vi "variant to tree helper.vi"(4 "is array element?":bool, 5 "is attribute?":bool, 6 "index string":string, 7 "name":string, 8 "error in (no error)":errorcluster, 9 "Item Indent":i32, 10 "Variant":variant, 11 "Items":T1(array[cluster])) -> (0 "error out":errorcluster, 3 "Items out":T1(array[cluster]))   [LabVIEW 2016]
uses:
  <vilib>/Utility/Data Type/NI_Data Type.lvlib
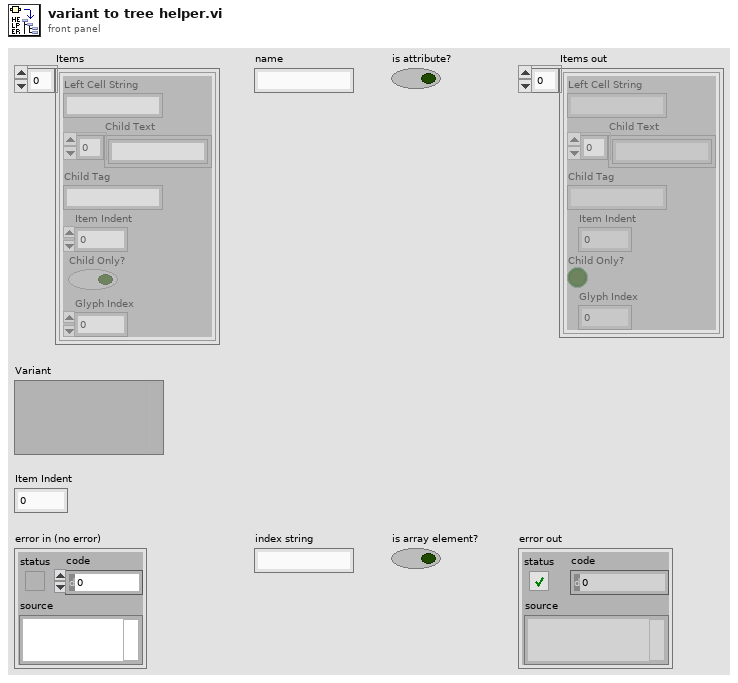
[diagram p1: front panel]
types:
  T1 = cluster{"Left Cell String":string, "Child Text":string[], "Child Tag":string, "Item Indent":i32, "Child Only?":bool, "Glyph Index":i32}[]
  T2 = typedef "NI_Data Type.lvlib/Data Type.ctl" = enum8{"Invalid Type", "Void", "I8", "I16", "I32", "I64", "U8", "U16", "U32", "U64", "Single Float", "Double Float", "Extended Float", "Single Complex", "Double Complex", "Extended Complex", "Enum U8", "Enum U16", "Enum U32", "Enum U64", "Single Float With Unit", "Double Float With Unit", "Extended Float With Unit", "Single Complex with Unit", "Double Complex with Unit", "Extended Complex with Unit", "Boolean", "String", "Path", "Picture", "Tag", "Array", "Cluster", "Variant", "LV Variant", "Waveform", "Timestamp", "Digital Waveform", "Digital Data", "ExpressData", "Refnum", "External Data", "VI", "Poly VI", "LabVIEW Class Instance", "Fixed Point"}
  T3 = cluster{"Left Cell String":string, "Child Text":string[], "Child Tag":string, "Item Indent":i32, "Child Only?":bool, "Glyph Index":i32}
  T4 = typedef "LVFixedPointRepRangeTypeDef.ctl" = cluster{"Range Min":dbl, "Range Max":dbl, "Delta":dbl}
  T5 = typedef "LVFixedPointRepBitsTypeDef.ctl" = cluster{"Signed":bool, "Word Length":u32, "Integer Word Length":i32}
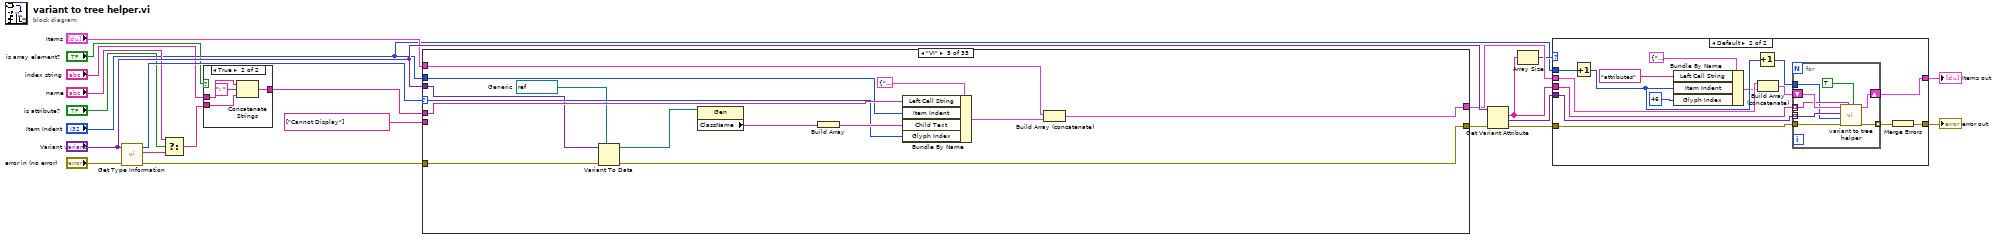
[diagram p0: block diagram]
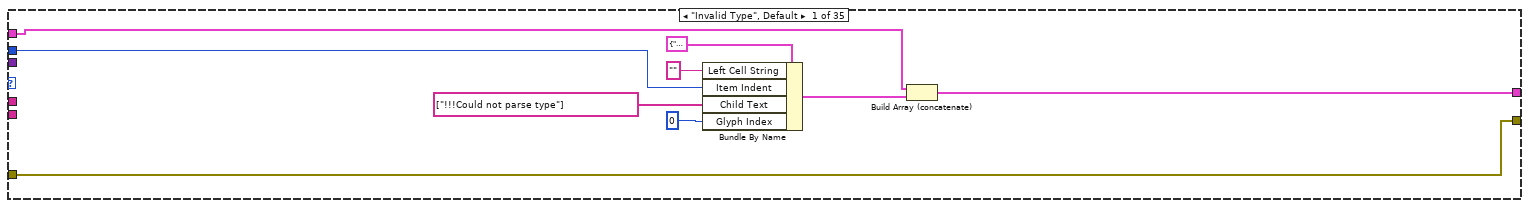
[diagram p4: hidden frame]
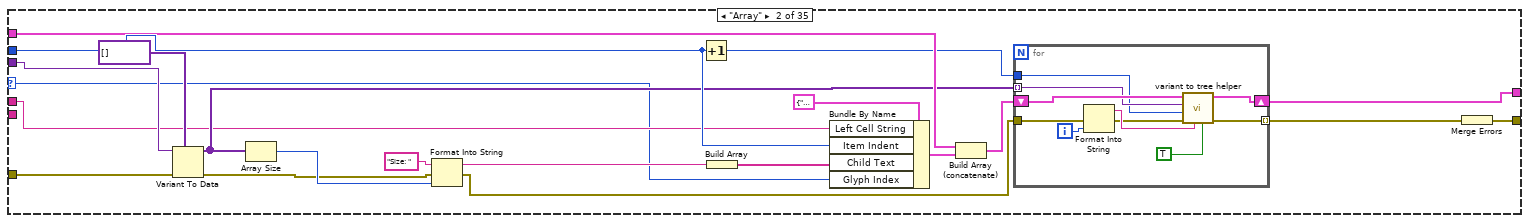
[diagram p5: hidden frame]
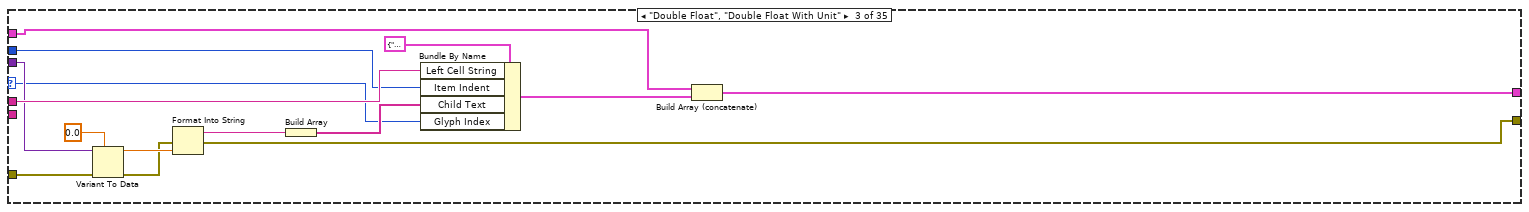
[diagram p6: hidden frame]
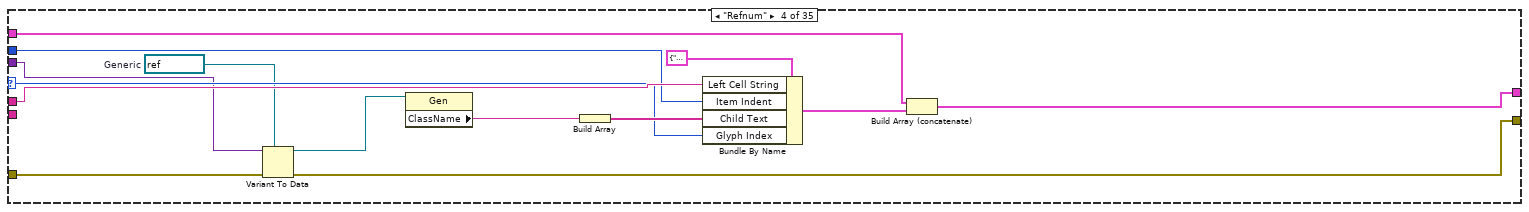
[diagram p7: hidden frame]
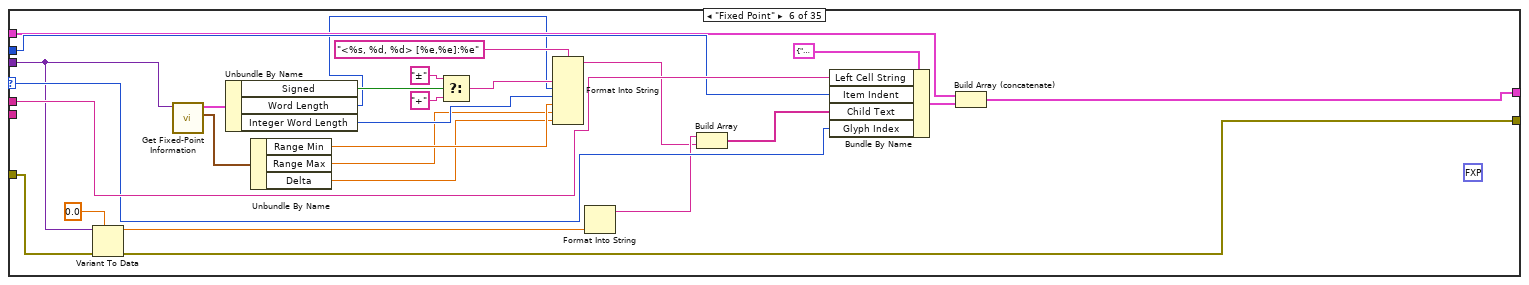
[diagram p8: hidden frame]
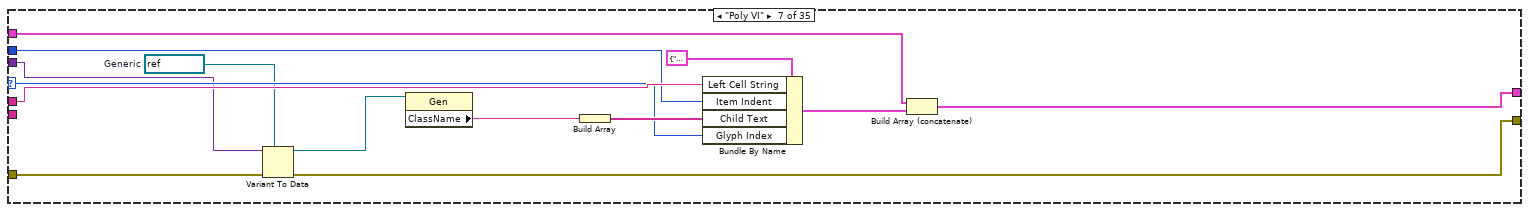
[diagram p9: hidden frame]
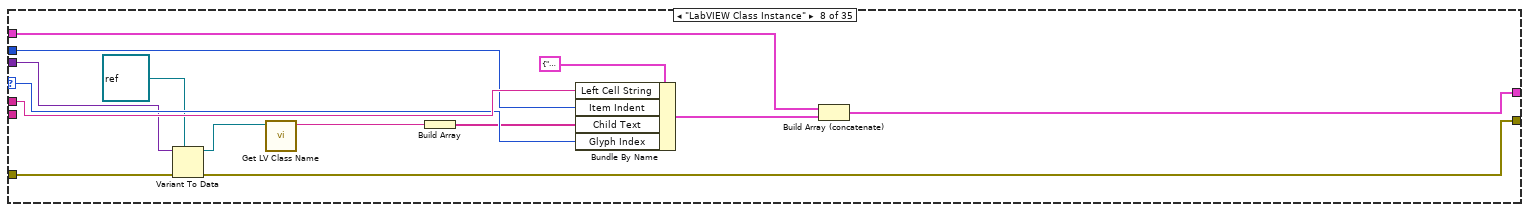
[diagram p10: hidden frame]
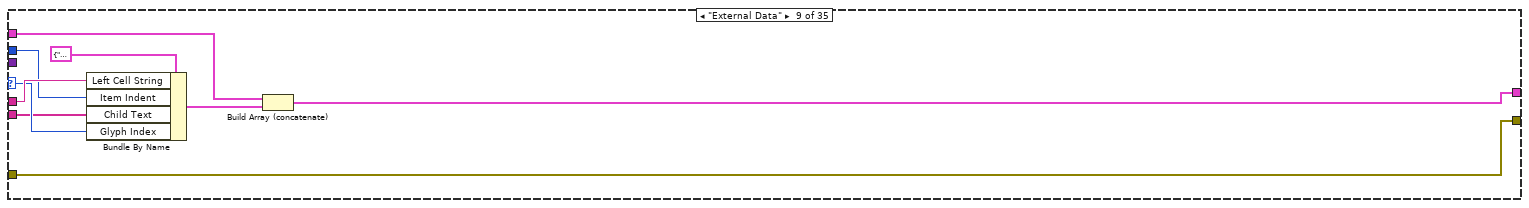
[diagram p11: hidden frame]
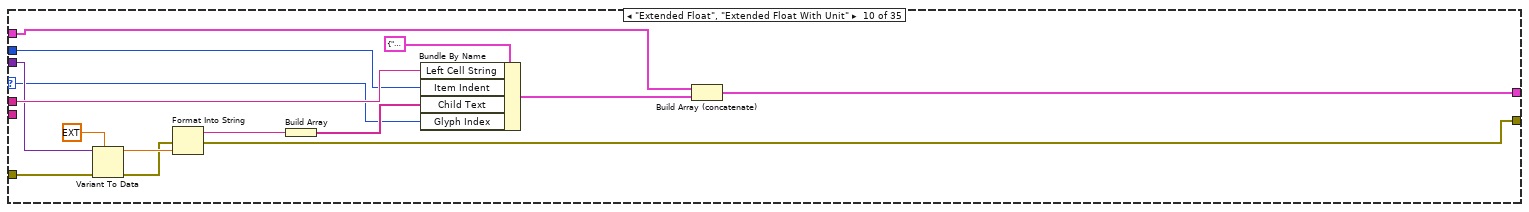
[diagram p12: hidden frame]
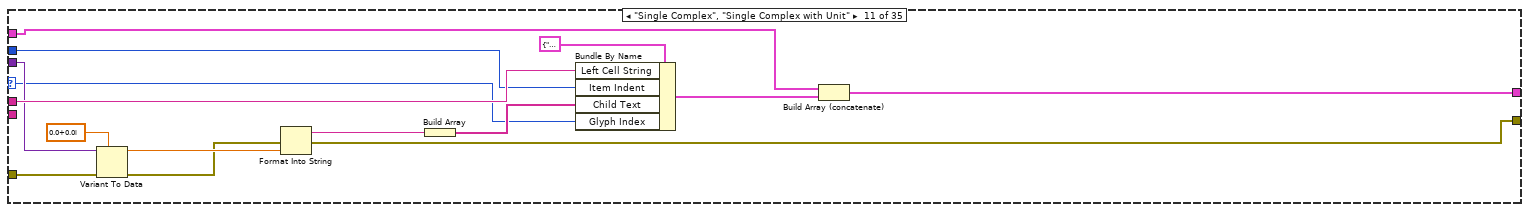
[diagram p13: hidden frame]
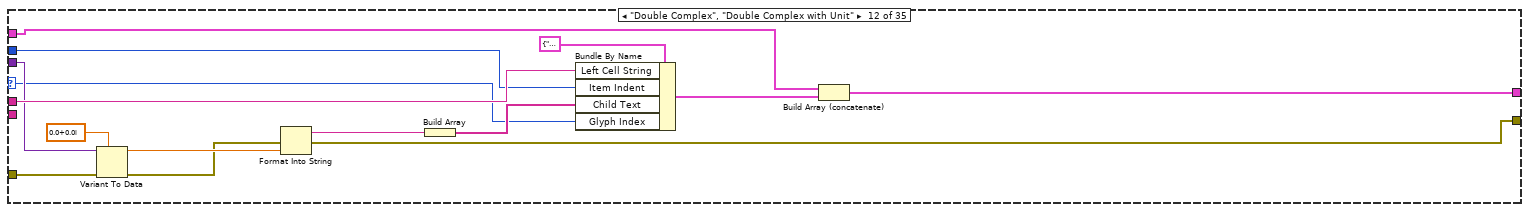
[diagram p14: hidden frame]
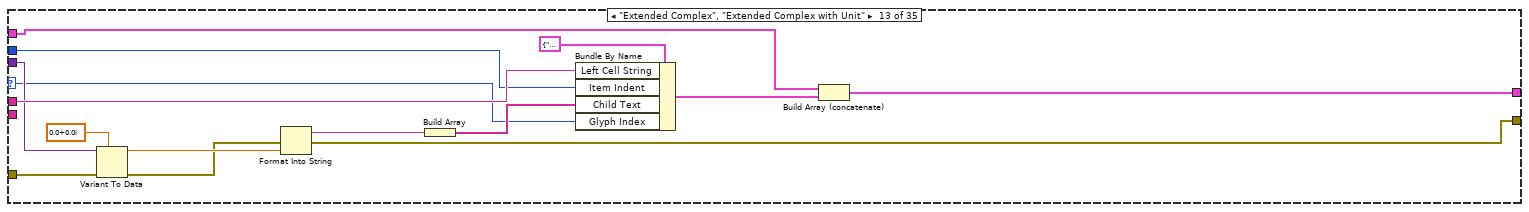
[diagram p15: hidden frame]
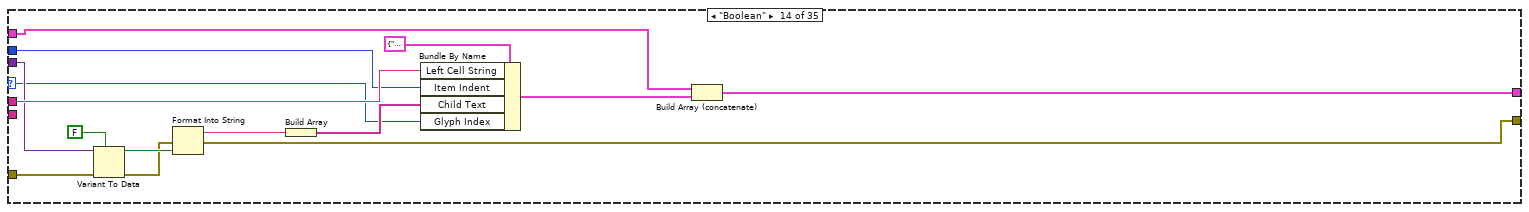
[diagram p16: hidden frame]
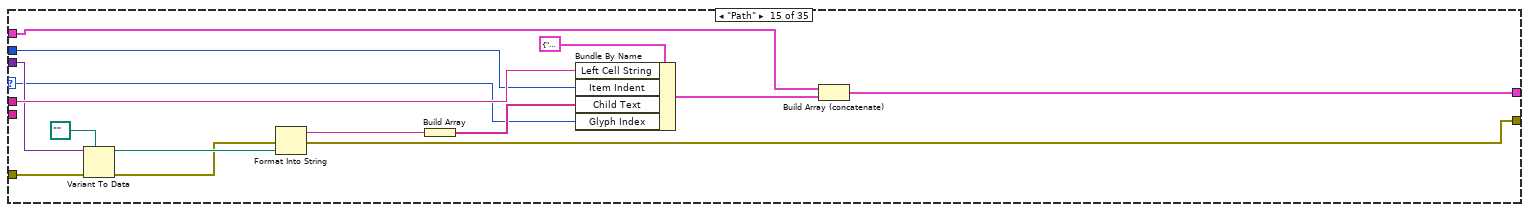
[diagram p17: hidden frame]
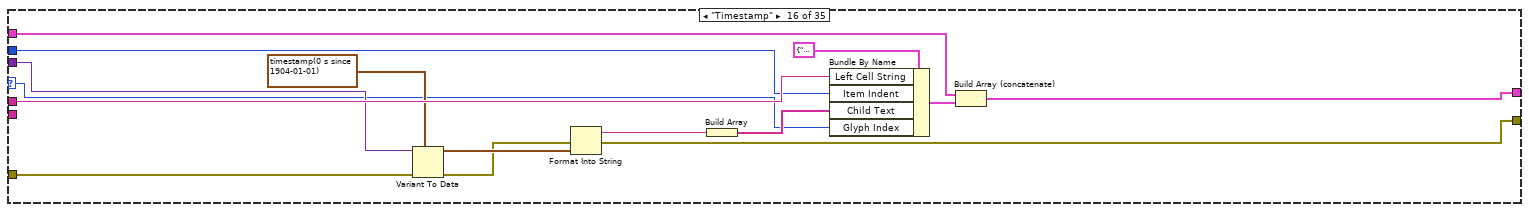
[diagram p18: hidden frame]
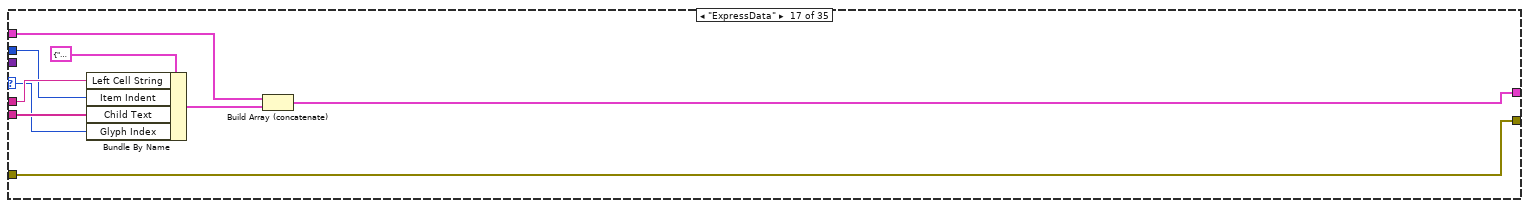
[diagram p19: hidden frame]
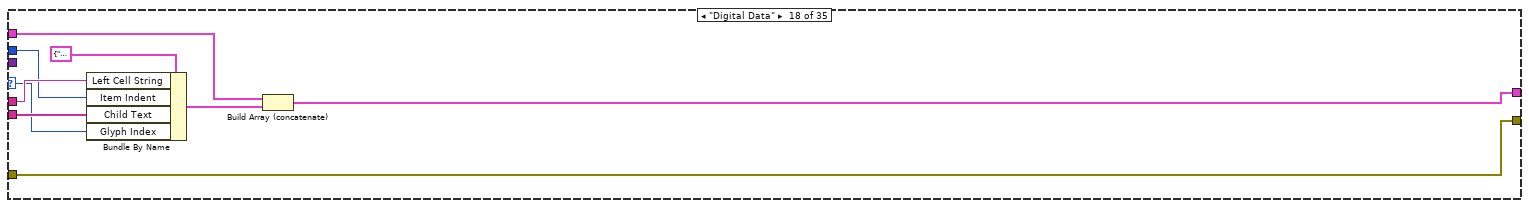
[diagram p20: hidden frame]
diagram:
  n1 = call <vilib>:"Get Type Information.vi"("error in (no error)"="error in (no error)", "Variant"="Variant") -> ("error out"=w4:errorcluster, "Name"=w14:string, "Type"=w22:T2)  [unwired: 5 in, 2 out]
  n2 = Select(t="name", s="is attribute?", f=w14) -> (s? t:f=w7:string)
  n3 = case shown="True" "is array element?" {
    tunnel: "index string" -> [_ w27]
    tunnel: w7 -> [w23 w25]
    tunnel: [w23 w24] -> w6
    frame False {
    }
    frame True {
      n4 = Concatenate Strings(w27, ": " ("string"), w25) -> (w24:string)
    }
  }
  n5 = case shown="\"VI\"" w22 {
    selector: w22 -> [_ w42 w71 w89 w103 w131 w144 w159 w168 w178 w193 w208 w223 w238 w253 w268 w281 w290 w299 w308 w317 w330 w361 w370 w380 w393 w409 w424 w439 w454 w469 w484 w499 w514 w529]
    tunnel: "Items" -> [w30 w53 w74 w92 w106 w134 w147 w162 w171 w181 w196 w211 w226 w241 w256 w271 w285 w294 w303 w313 w321 w344 w365 w374 w383 w401 w416 w431 w446 w461 w476 w491 w506 w521 w536]
    tunnel: "Variant" -> [_ w57 w79 w86 w100 w127 w141 w156 _ w186 w201 w216 w231 w246 w261 w276 _ _ _ _ _ w332 _ _ w387 w398 w413 w428 w443 w458 w473 w488 w503 w518 w533]
    tunnel: w6 -> [_ w43 w81 w95 w109 w136 w150 w164 w173 w188 w203 w218 w233 w248 w263 w278 w287 w296 w305 w314 w323 w345 w367 w376 w389 w404 w419 w434 w449 w464 w479 w494 w509 w524 w539]
    tunnel: "Item Indent" -> [w33 w54 w80 w94 w108 w135 w149 w163 w172 w187 w202 w217 w232 w247 w262 w277 w286 w295 w304 w309 w322 w339 w366 w375 w388 w403 w418 w433 w448 w463 w478 w493 w508 w523 w538]
    tunnel: [w28 w49 w72 w90 w104 w132 w145 w160 w169 w179 w194 w209 w224 w239 w254 w269 w283 w292 w301 w310 w319 w340 w363 w372 w381 w399 w414 w429 w444 w459 w474 w489 w504 w519 w534] -> w17
    tunnel: string[] ["Cannot Display"] ("Child Text") -> [_ _ _ _ _ _ _ _ w166 _ _ _ _ _ _ _ w282 w291 w300 w311 w318 _ w362 w371 _ _ _ _ _ _ _ _ _ _ _]
    tunnel: w4 -> [w36 w41 w70 w88 w102 w130 w143 w158 w167 w177 w192 w207 w222 w237 w252 w267 w280 w289 w298 w307 w316 w329 w360 w369 w379 w392 w408 w423 w438 w453 w468 w483 w498 w513 w528]
    tunnel: [w36 w37 w68 w87 w101 w129 w142 w157 w167 w175 w190 w205 w220 w235 w250 w265 w280 w289 w298 w307 w316 w325 w360 w369 w378 w391 w406 w421 w436 w451 w466 w481 w496 w511 w526] -> w1
    frame "Invalid Type", Default {
      n6 = Bundle By Name(cluster=T3 {"Left Cell String"="", "Child Text"=[], "Child Tag"="", "Item Indent"=0, "Child Only?"=FALSE, "Glyph Index"=0} ("Item"), "Left Cell String"="", "Item Indent"=w33, "Child Text"=string[] ["!!!Could not parse type"], "Glyph Index"=0) -> (w29:T3)
      n7 = Build Array (concatenate)(w30, w29) -> (w28:T1)
    }
    frame "Array" {
      n8 = Variant To Data(error in=w41, type=variant[] [], Variant=w57) -> (data=w47:variant[], error out=w40:errorcluster)
      n9 = Array Size(array=w47) -> (size(s)=w46:i32)
      n10 = Format Into String(initial string="Size: " ("string"), error in=w40, w46) -> (resulting string=w45:string, error out=w39:errorcluster)  [unwired: 1 in]
      n11 = Increment(x=w54) -> (x+1=w48:i32)
      n12 = Build Array(w45) -> (w51:string[])
      n13 = Bundle By Name(cluster=T3 {"Left Cell String"="", "Child Text"=[], "Child Tag"="", "Item Indent"=0, "Child Only?"=FALSE, "Glyph Index"=0} ("Item"), "Left Cell String"=w43, "Item Indent"=w54, "Child Text"=w51, "Glyph Index"=w42) -> (w52:T3)
      n14 = Build Array (concatenate)(w53, w52) -> (w50:T1)
      n15 = for {
        tunnel: w47 -> [w65] mode=indexing
        shift-right: [w66] -> w49
        shift-left: w50 -> [w67]
        tunnel: w48 -> [w64]
        tunnel: w39 -> [w60]
        tunnel: [w58] -> w38 mode=indexing
        i -> [w63]
        n16 = Format Into String(error in=w60, w63) -> (resulting string=w62:string, error out=w59:errorcluster)  [unwired: 2 in]
        n17 = call "variant to tree helper.vi"("is array element?"=TRUE, "index string"=w62, "error in (no error)"=w59, "Item Indent"=w64, "Variant"=w65, "Items"=w67) -> ("error out"=w58:errorcluster, "Items out"=w66:T1)  [unwired: 4 in]
      }
      n18 = Merge Errors(w38) -> (w37:errorcluster)
    }
    frame "Double Float", "Double Float With Unit" {
      n19 = Variant To Data(error in=w70, type=0.0, Variant=w79) -> (data=w77:dbl, error out=w69:errorcluster)
      n20 = Format Into String(error in=w69, w77) -> (resulting string=w76:string, error out=w68:errorcluster)  [unwired: 2 in]
      n21 = Build Array(w76) -> (w75:string[])
      n22 = Bundle By Name(cluster=T3 {"Left Cell String"="", "Child Text"=[], "Child Tag"="", "Item Indent"=0, "Child Only?"=FALSE, "Glyph Index"=0} ("Item"), "Left Cell String"=w81, "Item Indent"=w80, "Child Text"=w75, "Glyph Index"=w71) -> (w73:T3)
      n23 = Build Array (concatenate)(w74, w73) -> (w72:T1)
    }
    frame "Refnum" {
      w85 = refnum<vi> refnum  # Generic
      n24 = Variant To Data(error in=w88, type=w85, Variant=w86) -> (data=w84:refnum<vi>, error out=w87:errorcluster)
      n25 = property class="Gen"(reference=w84) -> ("ClassName"=w83:string)  [unwired: 1 in, 2 out]
      n26 = Build Array(w83) -> (w93:string[])
      n27 = Bundle By Name(cluster=T3 {"Left Cell String"="", "Child Text"=[], "Child Tag"="", "Item Indent"=0, "Child Only?"=FALSE, "Glyph Index"=0} ("Item"), "Left Cell String"=w95, "Item Indent"=w94, "Child Text"=w93, "Glyph Index"=w89) -> (w91:T3)
      n28 = Build Array (concatenate)(w92, w91) -> (w90:T1)
    }
    frame "VI" {
      w99 = refnum<vi> refnum  # Generic
      n29 = Variant To Data(error in=w102, type=w99, Variant=w100) -> (data=w98:refnum<vi>, error out=w101:errorcluster)
      n30 = property class="Gen"(reference=w98) -> ("ClassName"=w97:string)  [unwired: 1 in, 2 out]
      n31 = Build Array(w97) -> (w107:string[])
      n32 = Bundle By Name(cluster=T3 {"Left Cell String"="", "Child Text"=[], "Child Tag"="", "Item Indent"=0, "Child Only?"=FALSE, "Glyph Index"=0} ("Item"), "Left Cell String"=w109, "Item Indent"=w108, "Child Text"=w107, "Glyph Index"=w103) -> (w105:T3)
      n33 = Build Array (concatenate)(w106, w105) -> (w104:T1)
    }
    frame "Fixed Point" {
      (unwired) fxp<+,1,1> 0.0
      n34 = Variant To Data(error in=w130, type=0.0, Variant=w127) -> (data=w126:dbl, error out=w129:errorcluster)
      n35 = call <vilib>:"Get Fixed-Point Information.vi"("Variant"=w127) -> ("FXP Range"=w116:T4, "FXP Representation"=w123:T5)  [unwired: 7 in, 2 out]
      n36 = Unbundle By Name(w123) -> ("Signed"=w122:bool, "Word Length"=w118:u32, "Integer Word Length"=w117:i32)
      n37 = Unbundle By Name(w116) -> ("Range Min"=w115:dbl, "Range Max"=w114:dbl, "Delta"=w113:dbl)
      n38 = Select(t="±", s=w122, f="+" ("format string")) -> (s? t:f=w119:string)
      n39 = Format Into String(format string="<%s, %d, %d> [%e,%e]:%e", w119, w118, w117, w115, w114, w113) -> (resulting string=w111:string)  [unwired: 2 in, 1 out]
      n40 = Format Into String(w126) -> (resulting string=w125:string)  [unwired: 3 in, 1 out]
      n41 = Build Array(w125, w111) -> (w112:string[])
      n42 = Bundle By Name(cluster=T3 {"Left Cell String"="", "Child Text"=[], "Child Tag"="", "Item Indent"=0, "Child Only?"=FALSE, "Glyph Index"=0} ("Item"), "Left Cell String"=w136, "Item Indent"=w135, "Child Text"=w112, "Glyph Index"=w131) -> (w133:T3)
      n43 = Build Array (concatenate)(w134, w133) -> (w132:T1)
    }
    frame "Poly VI" {
      w140 = refnum<vi> refnum  # Generic
      n44 = Variant To Data(error in=w143, type=w140, Variant=w141) -> (data=w139:refnum<vi>, error out=w142:errorcluster)
      n45 = property class="Gen"(reference=w139) -> ("ClassName"=w138:string)  [unwired: 1 in, 2 out]
      n46 = Build Array(w138) -> (w148:string[])
      n47 = Bundle By Name(cluster=T3 {"Left Cell String"="", "Child Text"=[], "Child Tag"="", "Item Indent"=0, "Child Only?"=FALSE, "Glyph Index"=0} ("Item"), "Left Cell String"=w150, "Item Indent"=w149, "Child Text"=w148, "Glyph Index"=w144) -> (w146:T3)
      n48 = Build Array (concatenate)(w147, w146) -> (w145:T1)
    }
    frame "LabVIEW Class Instance" {
      n49 = Variant To Data(error in=w158, type=refnum<class> refnum ("LabVIEW Object"), Variant=w156) -> (data=w154:refnum<class>, error out=w157:errorcluster)
      n50 = call <vilib>:"Get LV Class Name.vi"("object"=w154) -> ("class name"=w153:string)  [unwired: 9 in, 1 out]
      n51 = Build Array(w153) -> (w152:string[])
      n52 = Bundle By Name(cluster=T3 {"Left Cell String"="", "Child Text"=[], "Child Tag"="", "Item Indent"=0, "Child Only?"=FALSE, "Glyph Index"=0} ("Item"), "Left Cell String"=w164, "Item Indent"=w163, "Child Text"=w152, "Glyph Index"=w159) -> (w161:T3)
      n53 = Build Array (concatenate)(w162, w161) -> (w160:T1)
    }
    frame "External Data" {
      n54 = Bundle By Name(cluster=T3 {"Left Cell String"="", "Child Text"=[], "Child Tag"="", "Item Indent"=0, "Child Only?"=FALSE, "Glyph Index"=0} ("Item"), "Left Cell String"=w173, "Item Indent"=w172, "Child Text"=w166, "Glyph Index"=w168) -> (w170:T3)
      n55 = Build Array (concatenate)(w171, w170) -> (w169:T1)
    }
    frame "Extended Float", "Extended Float With Unit" {
      n56 = Variant To Data(error in=w177, type=ext 0.0, Variant=w186) -> (data=w184:ext, error out=w176:errorcluster)
      n57 = Format Into String(error in=w176, w184) -> (resulting string=w183:string, error out=w175:errorcluster)  [unwired: 2 in]
      n58 = Build Array(w183) -> (w182:string[])
      n59 = Bundle By Name(cluster=T3 {"Left Cell String"="", "Child Text"=[], "Child Tag"="", "Item Indent"=0, "Child Only?"=FALSE, "Glyph Index"=0} ("Item"), "Left Cell String"=w188, "Item Indent"=w187, "Child Text"=w182, "Glyph Index"=w178) -> (w180:T3)
      n60 = Build Array (concatenate)(w181, w180) -> (w179:T1)
    }
    frame "Single Complex", "Single Complex with Unit" {
      n61 = Variant To Data(error in=w192, type=csg 0.0+0.0i, Variant=w201) -> (data=w199:csg, error out=w191:errorcluster)
      n62 = Format Into String(error in=w191, w199) -> (resulting string=w198:string, error out=w190:errorcluster)  [unwired: 2 in]
      n63 = Build Array(w198) -> (w197:string[])
      n64 = Bundle By Name(cluster=T3 {"Left Cell String"="", "Child Text"=[], "Child Tag"="", "Item Indent"=0, "Child Only?"=FALSE, "Glyph Index"=0} ("Item"), "Left Cell String"=w203, "Item Indent"=w202, "Child Text"=w197, "Glyph Index"=w193) -> (w195:T3)
      n65 = Build Array (concatenate)(w196, w195) -> (w194:T1)
    }
    frame "Double Complex", "Double Complex with Unit" {
      n66 = Variant To Data(error in=w207, type=cdb 0.0+0.0i, Variant=w216) -> (data=w214:cdb, error out=w206:errorcluster)
      n67 = Format Into String(error in=w206, w214) -> (resulting string=w213:string, error out=w205:errorcluster)  [unwired: 2 in]
      n68 = Build Array(w213) -> (w212:string[])
      n69 = Bundle By Name(cluster=T3 {"Left Cell String"="", "Child Text"=[], "Child Tag"="", "Item Indent"=0, "Child Only?"=FALSE, "Glyph Index"=0} ("Item"), "Left Cell String"=w218, "Item Indent"=w217, "Child Text"=w212, "Glyph Index"=w208) -> (w210:T3)
      n70 = Build Array (concatenate)(w211, w210) -> (w209:T1)
    }
    frame "Extended Complex", "Extended Complex with Unit" {
      n71 = Variant To Data(error in=w222, type=cdb 0.0+0.0i, Variant=w231) -> (data=w229:cdb, error out=w221:errorcluster)
      n72 = Format Into String(error in=w221, w229) -> (resulting string=w228:string, error out=w220:errorcluster)  [unwired: 2 in]
      n73 = Build Array(w228) -> (w227:string[])
      n74 = Bundle By Name(cluster=T3 {"Left Cell String"="", "Child Text"=[], "Child Tag"="", "Item Indent"=0, "Child Only?"=FALSE, "Glyph Index"=0} ("Item"), "Left Cell String"=w233, "Item Indent"=w232, "Child Text"=w227, "Glyph Index"=w223) -> (w225:T3)
      n75 = Build Array (concatenate)(w226, w225) -> (w224:T1)
    }
    frame "Boolean" {
      n76 = Variant To Data(error in=w237, type=FALSE, Variant=w246) -> (data=w244:bool, error out=w236:errorcluster)
      n77 = Format Into String(error in=w236, w244) -> (resulting string=w243:string, error out=w235:errorcluster)  [unwired: 2 in]
      n78 = Build Array(w243) -> (w242:string[])
      n79 = Bundle By Name(cluster=T3 {"Left Cell String"="", "Child Text"=[], "Child Tag"="", "Item Indent"=0, "Child Only?"=FALSE, "Glyph Index"=0} ("Item"), "Left Cell String"=w248, "Item Indent"=w247, "Child Text"=w242, "Glyph Index"=w238) -> (w240:T3)
      n80 = Build Array (concatenate)(w241, w240) -> (w239:T1)
    }
    frame "Path" {
      n81 = Variant To Data(error in=w252, type=path "", Variant=w261) -> (data=w259:path, error out=w251:errorcluster)
      n82 = Format Into String(error in=w251, w259) -> (resulting string=w258:string, error out=w250:errorcluster)  [unwired: 2 in]
      n83 = Build Array(w258) -> (w257:string[])
      n84 = Bundle By Name(cluster=T3 {"Left Cell String"="", "Child Text"=[], "Child Tag"="", "Item Indent"=0, "Child Only?"=FALSE, "Glyph Index"=0} ("Item"), "Left Cell String"=w263, "Item Indent"=w262, "Child Text"=w257, "Glyph Index"=w253) -> (w255:T3)
      n85 = Build Array (concatenate)(w256, w255) -> (w254:T1)
    }
    frame "Timestamp" {
      n86 = Variant To Data(error in=w267, type=timestamp(0 s since 1904-01-01) ("Time Stamp"), Variant=w276) -> (data=w274:timestamp, error out=w266:errorcluster)
      n87 = Format Into String(error in=w266, w274) -> (resulting string=w273:string, error out=w265:errorcluster)  [unwired: 2 in]
      n88 = Build Array(w273) -> (w272:string[])
      n89 = Bundle By Name(cluster=T3 {"Left Cell String"="", "Child Text"=[], "Child Tag"="", "Item Indent"=0, "Child Only?"=FALSE, "Glyph Index"=0} ("Item"), "Left Cell String"=w278, "Item Indent"=w277, "Child Text"=w272, "Glyph Index"=w268) -> (w270:T3)
      n90 = Build Array (concatenate)(w271, w270) -> (w269:T1)
    }
    frame "ExpressData" {
      n91 = Bundle By Name(cluster=T3 {"Left Cell String"="", "Child Text"=[], "Child Tag"="", "Item Indent"=0, "Child Only?"=FALSE, "Glyph Index"=0} ("Item"), "Left Cell String"=w287, "Item Indent"=w286, "Child Text"=w282, "Glyph Index"=w281) -> (w284:T3)
      n92 = Build Array (concatenate)(w285, w284) -> (w283:T1)
    }
    frame "Digital Data" {
      n93 = Bundle By Name(cluster=T3 {"Left Cell String"="", "Child Text"=[], "Child Tag"="", "Item Indent"=0, "Child Only?"=FALSE, "Glyph Index"=0} ("Item"), "Left Cell String"=w296, "Item Indent"=w295, "Child Text"=w291, "Glyph Index"=w290) -> (w293:T3)
      n94 = Build Array (concatenate)(w294, w293) -> (w292:T1)
    }
    frame "Digital Waveform" {
      n95 = Bundle By Name(cluster=T3 {"Left Cell String"="", "Child Text"=[], "Child Tag"="", "Item Indent"=0, "Child Only?"=FALSE, "Glyph Index"=0} ("Item"), "Left Cell String"=w305, "Item Indent"=w304, "Child Text"=w300, "Glyph Index"=w299) -> (w302:T3)
      n96 = Build Array (concatenate)(w303, w302) -> (w301:T1)
    }
    frame "Void", "Variant", "LV Variant" {
      n97 = Bundle By Name(cluster=T3 {"Left Cell String"="", "Child Text"=[], "Child Tag"="", "Item Indent"=0, "Child Only?"=FALSE, "Glyph Index"=0} ("Item"), "Left Cell String"=w314, "Item Indent"=w309, "Child Text"=w311, "Glyph Index"=w308) -> (w312:T3)
      n98 = Build Array (concatenate)(w313, w312) -> (w310:T1)
    }
    frame "Waveform" {
      n99 = Bundle By Name(cluster=T3 {"Left Cell String"="", "Child Text"=[], "Child Tag"="", "Item Indent"=0, "Child Only?"=FALSE, "Glyph Index"=0} ("Item"), "Left Cell String"=w323, "Item Indent"=w322, "Child Text"=w318, "Glyph Index"=w317) -> (w320:T3)
      n100 = Build Array (concatenate)(w321, w320) -> (w319:T1)
    }
    frame "Cluster" {
      n101 = Variant To Flattened String(Variant=w332) -> (data string=w342:string)  [unwired: 1 out]
      n102 = call <vilib>:"Get Cluster Information.vi"("error in (no error)"=w329, "Variant"=w332) -> ("error out"=w328:errorcluster, "Cluster Elements"=w331:variant[])  [unwired: 8 in]
      n103 = for {
        tunnel: w331 -> [w359] mode=indexing
        tunnel: [w357] -> w337 mode=indexing
        shift-right: [w353] -> _
        shift-left: w342 -> [w356]
        n104 = Variant To Flattened String(Variant=w359) -> (1:w358:i16[])  [unwired: 1 out]
        n105 = Flattened String To Variant(6:w356, 7:w358) -> (3:w357:variant)  [unwired: 1 in, 1 out]
        n106 = Variant To Flattened String(Variant=w357) -> (data string=w355:string)  [unwired: 1 out]
        n107 = String Length(string=w355) -> (length=w354:i32)
        n108 = String Subset(string=w356, offset (0)=w354) -> (substring=w353:string)  [unwired: 1 in]
      }
      n109 = Increment(x=w339) -> (x+1=w338:i32)
      n110 = Array Size(array=w337) -> (size(s)=w336:i32)
      n111 = Format Into String(initial string="Number of Elements: ", error in=w328, w336) -> (resulting string=w334:string, error out=w327:errorcluster)  [unwired: 1 in]
      n112 = Build Array(w334) -> (w333:string[])
      n113 = Bundle By Name(cluster=T3 {"Left Cell String"="", "Child Text"=[], "Child Tag"="", "Item Indent"=0, "Child Only?"=FALSE, "Glyph Index"=0} ("Item"), "Left Cell String"=w345, "Item Indent"=w339, "Child Text"=w333, "Glyph Index"=w330) -> (w343:T3)
      n114 = Build Array (concatenate)(w344, w343) -> (w341:T1)
      n115 = for {
        tunnel: w337 -> [w351] mode=indexing
        shift-right: [w350] -> w340
        shift-left: w341 -> [w352]
        tunnel: w338 -> [w349]
        tunnel: w327 -> [w348]
        tunnel: [w347] -> w326 mode=indexing
        n116 = call "variant to tree helper.vi"("error in (no error)"=w348, "Item Indent"=w349, "Variant"=w351, "Items"=w352) -> ("error out"=w347:errorcluster, "Items out"=w350:T1)  [unwired: 6 in]
      }
      n117 = Merge Errors(w326) -> (w325:errorcluster)
    }
    frame "Tag" {
      n118 = Bundle By Name(cluster=T3 {"Left Cell String"="", "Child Text"=[], "Child Tag"="", "Item Indent"=0, "Child Only?"=FALSE, "Glyph Index"=0} ("Item"), "Left Cell String"=w367, "Item Indent"=w366, "Child Text"=w362, "Glyph Index"=w361) -> (w364:T3)
      n119 = Build Array (concatenate)(w365, w364) -> (w363:T1)
    }
    frame "Picture" {
      n120 = Bundle By Name(cluster=T3 {"Left Cell String"="", "Child Text"=[], "Child Tag"="", "Item Indent"=0, "Child Only?"=FALSE, "Glyph Index"=0} ("Item"), "Left Cell String"=w376, "Item Indent"=w375, "Child Text"=w371, "Glyph Index"=w370) -> (w373:T3)
      n121 = Build Array (concatenate)(w374, w373) -> (w372:T1)
    }
    frame "String" {
      n122 = Variant To Data(error in=w379, type="", Variant=w387) -> (data=w385:string, error out=w378:errorcluster)
      n123 = Build Array(w385) -> (w384:string[])
      n124 = Bundle By Name(cluster=T3 {"Left Cell String"="", "Child Text"=[], "Child Tag"="", "Item Indent"=0, "Child Only?"=FALSE, "Glyph Index"=0} ("Item"), "Left Cell String"=w389, "Item Indent"=w388, "Child Text"=w384, "Glyph Index"=w380) -> (w382:T3)
      n125 = Build Array (concatenate)(w383, w382) -> (w381:T1)
    }
    frame "Enum U8".."Enum U64" {
      n126 = call <vilib>:"Get Numeric Information.vi"("Variant"=w398) -> ("Enum Names"=w397:string[])  [unwired: 7 in, 3 out]
      n127 = Variant To Data(error in=w392, type=u64 0, Variant=w398) -> (data=w394:u64, error out=w391:errorcluster)
      n128 = Index Array(array=w397, index=w394) -> (element=w396:string)
      n129 = Build Array(w396) -> (w395:string[])
      n130 = Bundle By Name(cluster=T3 {"Left Cell String"="", "Child Text"=[], "Child Tag"="", "Item Indent"=0, "Child Only?"=FALSE, "Glyph Index"=0} ("Item"), "Left Cell String"=w404, "Item Indent"=w403, "Child Text"=w395, "Glyph Index"=w393) -> (w400:T3)
      n131 = Build Array (concatenate)(w401, w400) -> (w399:T1)
    }
    frame "Single Float", "Single Float With Unit" {
      n132 = Variant To Data(error in=w408, type=sgl 0.0, Variant=w413) -> (data=w412:sgl, error out=w407:errorcluster)
      n133 = Format Into String(error in=w407, w412) -> (resulting string=w410:string, error out=w406:errorcluster)  [unwired: 2 in]
      n134 = Build Array(w410) -> (w411:string[])
      n135 = Bundle By Name(cluster=T3 {"Left Cell String"="", "Child Text"=[], "Child Tag"="", "Item Indent"=0, "Child Only?"=FALSE, "Glyph Index"=0} ("Item"), "Left Cell String"=w419, "Item Indent"=w418, "Child Text"=w411, "Glyph Index"=w409) -> (w415:T3)
      n136 = Build Array (concatenate)(w416, w415) -> (w414:T1)
    }
    frame "I8" {
      n137 = Variant To Data(error in=w423, type=i8 0, Variant=w428) -> (data=w427:i8, error out=w422:errorcluster)
      n138 = Format Into String(error in=w422, w427) -> (resulting string=w425:string, error out=w421:errorcluster)  [unwired: 2 in]
      n139 = Build Array(w425) -> (w426:string[])
      n140 = Bundle By Name(cluster=T3 {"Left Cell String"="", "Child Text"=[], "Child Tag"="", "Item Indent"=0, "Child Only?"=FALSE, "Glyph Index"=0} ("Item"), "Left Cell String"=w434, "Item Indent"=w433, "Child Text"=w426, "Glyph Index"=w424) -> (w430:T3)
      n141 = Build Array (concatenate)(w431, w430) -> (w429:T1)
    }
    frame "I16" {
      n142 = Variant To Data(error in=w438, type=i16 0, Variant=w443) -> (data=w442:i16, error out=w437:errorcluster)
      n143 = Format Into String(error in=w437, w442) -> (resulting string=w440:string, error out=w436:errorcluster)  [unwired: 2 in]
      n144 = Build Array(w440) -> (w441:string[])
      n145 = Bundle By Name(cluster=T3 {"Left Cell String"="", "Child Text"=[], "Child Tag"="", "Item Indent"=0, "Child Only?"=FALSE, "Glyph Index"=0} ("Item"), "Left Cell String"=w449, "Item Indent"=w448, "Child Text"=w441, "Glyph Index"=w439) -> (w445:T3)
      n146 = Build Array (concatenate)(w446, w445) -> (w444:T1)
    }
    frame "I32" {
      n147 = Variant To Data(error in=w453, type=0, Variant=w458) -> (data=w457:i32, error out=w452:errorcluster)
      n148 = Format Into String(error in=w452, w457) -> (resulting string=w455:string, error out=w451:errorcluster)  [unwired: 2 in]
      n149 = Build Array(w455) -> (w456:string[])
      n150 = Bundle By Name(cluster=T3 {"Left Cell String"="", "Child Text"=[], "Child Tag"="", "Item Indent"=0, "Child Only?"=FALSE, "Glyph Index"=0} ("Item"), "Left Cell String"=w464, "Item Indent"=w463, "Child Text"=w456, "Glyph Index"=w454) -> (w460:T3)
      n151 = Build Array (concatenate)(w461, w460) -> (w459:T1)
    }
    frame "I64" {
      n152 = Variant To Data(error in=w468, type=i64 0, Variant=w473) -> (data=w472:i64, error out=w467:errorcluster)
      n153 = Format Into String(error in=w467, w472) -> (resulting string=w470:string, error out=w466:errorcluster)  [unwired: 2 in]
      n154 = Build Array(w470) -> (w471:string[])
      n155 = Bundle By Name(cluster=T3 {"Left Cell String"="", "Child Text"=[], "Child Tag"="", "Item Indent"=0, "Child Only?"=FALSE, "Glyph Index"=0} ("Item"), "Left Cell String"=w479, "Item Indent"=w478, "Child Text"=w471, "Glyph Index"=w469) -> (w475:T3)
      n156 = Build Array (concatenate)(w476, w475) -> (w474:T1)
    }
    frame "U8" {
      n157 = Variant To Data(error in=w483, type=u8 0, Variant=w488) -> (data=w487:u8, error out=w482:errorcluster)
      n158 = Format Into String(error in=w482, w487) -> (resulting string=w485:string, error out=w481:errorcluster)  [unwired: 2 in]
      n159 = Build Array(w485) -> (w486:string[])
      n160 = Bundle By Name(cluster=T3 {"Left Cell String"="", "Child Text"=[], "Child Tag"="", "Item Indent"=0, "Child Only?"=FALSE, "Glyph Index"=0} ("Item"), "Left Cell String"=w494, "Item Indent"=w493, "Child Text"=w486, "Glyph Index"=w484) -> (w490:T3)
      n161 = Build Array (concatenate)(w491, w490) -> (w489:T1)
    }
    frame "U16" {
      n162 = Variant To Data(error in=w498, type=u16 0, Variant=w503) -> (data=w502:u16, error out=w497:errorcluster)
      n163 = Format Into String(error in=w497, w502) -> (resulting string=w500:string, error out=w496:errorcluster)  [unwired: 2 in]
      n164 = Build Array(w500) -> (w501:string[])
      n165 = Bundle By Name(cluster=T3 {"Left Cell String"="", "Child Text"=[], "Child Tag"="", "Item Indent"=0, "Child Only?"=FALSE, "Glyph Index"=0} ("Item"), "Left Cell String"=w509, "Item Indent"=w508, "Child Text"=w501, "Glyph Index"=w499) -> (w505:T3)
      n166 = Build Array (concatenate)(w506, w505) -> (w504:T1)
    }
    frame "U32" {
      n167 = Variant To Data(error in=w513, type=u32 0, Variant=w518) -> (data=w517:u32, error out=w512:errorcluster)
      n168 = Format Into String(error in=w512, w517) -> (resulting string=w515:string, error out=w511:errorcluster)  [unwired: 2 in]
      n169 = Build Array(w515) -> (w516:string[])
      n170 = Bundle By Name(cluster=T3 {"Left Cell String"="", "Child Text"=[], "Child Tag"="", "Item Indent"=0, "Child Only?"=FALSE, "Glyph Index"=0} ("Item"), "Left Cell String"=w524, "Item Indent"=w523, "Child Text"=w516, "Glyph Index"=w514) -> (w520:T3)
      n171 = Build Array (concatenate)(w521, w520) -> (w519:T1)
    }
    frame "U64" {
      n172 = Variant To Data(error in=w528, type=u64 0, Variant=w533) -> (data=w532:u64, error out=w527:errorcluster)
      n173 = Format Into String(error in=w527, w532) -> (resulting string=w530:string, error out=w526:errorcluster)  [unwired: 2 in]
      n174 = Build Array(w530) -> (w531:string[])
      n175 = Bundle By Name(cluster=T3 {"Left Cell String"="", "Child Text"=[], "Child Tag"="", "Item Indent"=0, "Child Only?"=FALSE, "Glyph Index"=0} ("Item"), "Left Cell String"=w539, "Item Indent"=w538, "Child Text"=w531, "Glyph Index"=w529) -> (w535:T3)
      n176 = Build Array (concatenate)(w536, w535) -> (w534:T1)
    }
  }
  n177 = Get Variant Attribute(Variant="Variant", error in=w1) -> (names=w13:string[], values=w19:variant[], error out=w3:errorcluster)  [unwired: 2 in, 1 out]
  n178 = Array Size(array=w13) -> (size(s)=w12:i32)
  n179 = case shown="Default" w12 {
    tunnel: w19 -> [_ w557]
    tunnel: w17 -> [w542 w554]
    tunnel: [w542 w556] -> w16
    tunnel: w13 -> [_ w555]
    tunnel: "Item Indent" -> [_ w553]
    tunnel: w3 -> [w541 w545]
    tunnel: [w541 w543] -> w2
    frame 0 {
    }
    frame Default {
      n180 = Increment(x=w553) -> (x+1=w549:i32)
      n181 = Bundle By Name(cluster=T3 {"Left Cell String"="", "Child Text"=[], "Child Tag"="", "Item Indent"=0, "Child Only?"=FALSE, "Glyph Index"=0} ("Item"), "Left Cell String"="attributes", "Item Indent"=w549, "Glyph Index"=46) -> (w548:T3)
      n182 = Increment(x=w549) -> (x+1=w552:i32)
      n183 = Build Array (concatenate)(w554, w548) -> (w547:T1)
      n184 = for {
        tunnel: w557 -> [w565] mode=indexing
        shift-right: [w563] -> w556
        shift-left: w547 -> [w564]
        tunnel: w555 -> [w562] mode=indexing
        tunnel: w552 -> [w560]
        tunnel: w545 -> [w559]
        tunnel: [w558] -> w544 mode=indexing
        n185 = call "variant to tree helper.vi"("is attribute?"=TRUE, "name"=w562, "error in (no error)"=w559, "Item Indent"=w560, "Variant"=w565, "Items"=w564) -> ("error out"=w558:errorcluster, "Items out"=w563:T1)  [unwired: 4 in]
      }
      n186 = Merge Errors(w544) -> (w543:errorcluster)
    }
  }
  "Items out" <- w16
  "error out" <- w2
